vi "MsgStopSync.vi"   [LabVIEW 2018]
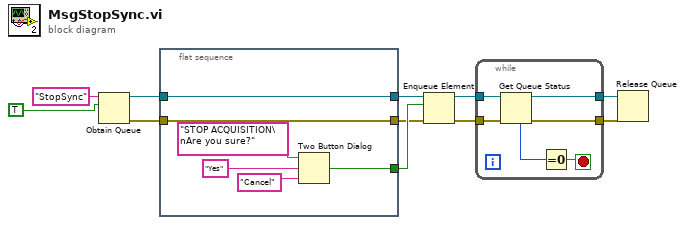
[diagram p0: block diagram]
diagram:
  n1 = Obtain Queue(name (unnamed)="StopSync", element data type=TRUE) -> (queue out=w9:refnum<queue>, error out=w6:errorcluster)  [unwired: 3 in, 1 out]
  n2 = flat-sequence {
    tunnel: w9 -> [w14]
    tunnel: [w14] -> w8
    tunnel: [w13] -> w7
    tunnel: [w12] -> w5
    tunnel: w6 -> [w12]
    frame #0 {
      n3 = Two Button Dialog(message="STOP ACQUISITION\nAre you sure?", 1:"Cancel" ("F button name (\"Cancel\")"), 2:"Yes" ("T button name (\"OK\")")) -> (T button?=w13:bool)
    }
  }
  n4 = Enqueue Element(queue=w8, element=w7, error in (no error)=w5) -> (queue out=w4:refnum<queue>, error out=w3:errorcluster)  [unwired: 1 in, 1 out]
  n5 = while {
    tunnel: w4 -> [w23]
    tunnel: w3 -> [w22]
    tunnel: [w21] -> w2
    tunnel: [w20] -> w1
    stop <- w19 stop-if-true
    n6 = Get Queue Status(queue=w23, error in (no error)=w22) -> (queue out=w21:refnum<queue>, error out=w20:errorcluster, # elements in queue=w18:i32)  [unwired: 1 in, 5 out]
    n7 = Equal To 0?(x=w18) -> (x = 0?=w19:bool)
  }
  n8 = Release Queue(queue=w2, error in (no error)=w1) -> ()  [unwired: 1 in, 3 out]
